vi "All Control Types in Memory.vi"() -> (2 "Control Types":T1(c390))   [LabVIEW 2020, in "VolatusControl.lvlib" / "DigitalControlModule.lvclass"]
uses:
  DigitalControlModule.lvclass
  DigitalControlModule.lvclass/DigitalControlModule.ctl
  DigitalControl/DigitalControl.lvclass
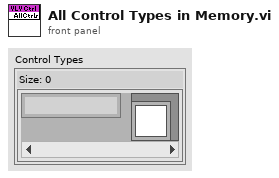
[diagram p1: front panel]
types:
  T1 = map{string, refnum<class "DigitalControl.lvclass">}
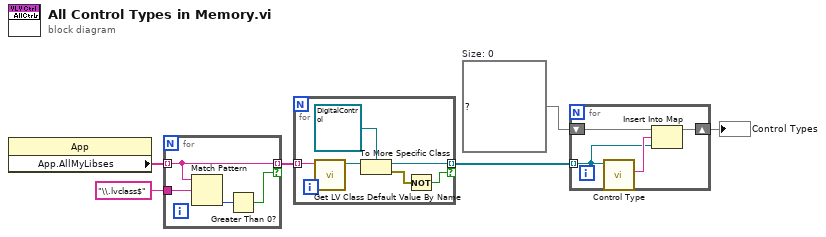
[diagram p0: block diagram]
diagram:
  w2 = T1 {}  # Size: 0
  n1 = property class="App"() -> ("App.AllMyLibses"=w6:string[])  [unwired: 2 in, 2 out]
  n2 = for {
    tunnel: w6 -> [w10] mode=indexing
    tunnel: [w10] -> w4 mode=indexing if=w7
    tunnel: "\\.lvclass$" -> [w9]
    n3 = Match Pattern(string=w10, regular expression=w9) -> (offset past match=w8:i32)  [unwired: 1 in, 3 out]
    n4 = Greater Than 0?(x=w8) -> (x > 0?=w7:bool)
  }
  n5 = for {
    tunnel: w4 -> [w16] mode=indexing
    tunnel: [w13] -> w3 mode=indexing if=w11
    n6 = call <vilib>:"Get LV Class Default Value By Name.vi"("class name"=w16) -> ("object"=w15:refnum<class>)  [unwired: 9 in, 1 out]
    n7 = To More Specific Class(target class=refnum<class "DigitalControl.lvclass"> refnum ("VolatusControl.lvlib:ValveControl.lvclass"), reference=w15) -> (specific class reference=w13:refnum<class "DigitalControl.lvclass">, error out=w12:errorcluster)  [unwired: 1 in]
    n8 = Not(x=w12) -> (.not. x?=w11:bool)
  }
  n9 = for {
    tunnel: w3 -> [w17] mode=indexing
    shift-right: [w18] -> w1
    shift-left: w2 -> [w20]
    n10 = call-dynamic "Control Type.vi"("Valve in"=w17) -> ("Valve Type"=w19:string)  [unwired: 10 in]
    n11 = Insert Into Map(map in=w20, key=w19, value=w17) -> (map out=w18:T1)  [unwired: 2 out]
  }
  "Control Types" <- w1
